vi "PCO_SetApertureF.vi"(8 "error in (no error)":errorcluster {"code" format="%x"}, 9 "dwflagsin":u32, 10 "dwfAperturePos":u32, 11 "hLens":u64) -> (0 "error out":errorcluster {"code" format="%x"}, 1 "dwfAperturePos out":u32, 2 "ErrorMessage":i32 format="%x", 3 "hLens out":u64, 5 "dwflagsout":u32)   [LabVIEW 2019, in "SDK.lvlib" / "LensControl.lvlib"]
doc: "<b>Description:</b>\nSets the current aperture position of the lens control device in f/position * 10 (member of dwApertures)\nPlease select a member of the current dwApertures array.\nThe dwApertures array is reinitialized in case the zoom changes and either PCO_GetApertureF or PCO_SetApertureF are called.\nChange in zoom will be shown in dwflagsout as LENSCONTROL_OUT_ZOOMHASCHANGED.\n\n<b>Supported camera type:</b>\npco.edge CLHS, pco.dimax cs\n\n<b>Descriptor dependency:</b>\nNone"
uses:
  LensControl.lvlib
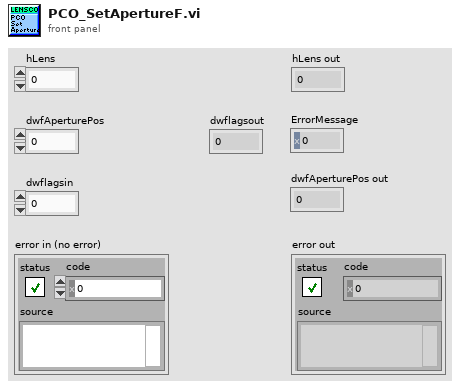
[diagram p1: front panel]
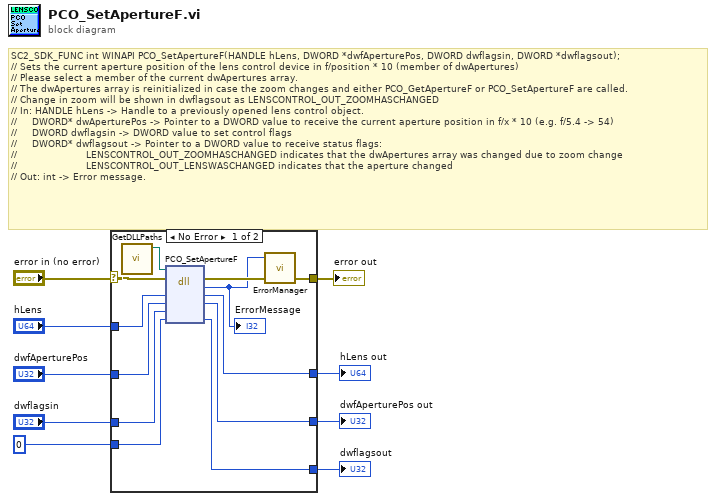
[diagram p0: block diagram]
diagram:
  # "SC2_SDK_FUNC int WINAPI PCO_SetApertureF(HANDLE hLens, DWORD *dwfAperturePos, DWORD dwflagsin, DWORD *dwflagsout);\n// Sets the current aperture position of the lens control device in f/position * 10 (member of dwApertures)\n// Please select a member of the current dwApertures array.\n// The dwApertures array is reinitialized in case the zoom changes and either PCO_GetApertureF or PCO_SetApertureF are called.\n// Change in zoom will be shown in dwflagsout as LENSCONTROL_OUT_ZOOMHASCHANGED\n// In: HANDLE hLens -> Handle to a previously opened lens control object.\n//     DWORD* dwAperturePos -> Pointer to a DWORD value to receive the current aperture position in f/x * 10 (e.g. f/5.4 -> 54)\n//     DWORD dwflagsin -> DWORD value to set control flags\n//     DWORD* dwflagsout -> Pointer to a DWORD value to receive status flags:\n//                       LENSCONTROL_OUT_ZOOMHASCHANGED indicates that the dwApertures array was changed due to zoom change\n//                       LENSCONTROL_OUT_LENSWASCHANGED indicates that the aperture changed\n// Out: int -> Error message."
  n1 = case shown="No Error" "error in (no error)" {
    selector: "error in (no error)" -> [w14 w22]
    tunnel: "hLens" -> [w21 w25]
    tunnel: [w20 w25] -> w8
    tunnel: "dwfAperturePos" -> [w19 w24]
    tunnel: [w18 w24] -> w6
    tunnel: "dwflagsin" -> [w17 _]
    tunnel: u32 0 ("dwflagsout") -> [w16 w23]
    tunnel: [w15 w23] -> w3
    tunnel: [w13 w22] -> w2
    frame No Error {
      n2 = call "GetDLLPaths.vi"() -> ("SC2_Cam_Path"=w10:path)  [unwired: 8 in, 3 out]
      n3 = dll-call lib="?" fn="PCO_SetApertureF"(path in=w10, error in=w14, "hLens"=w21, "dwfAperturePos"=w19, "dwflagsin"=w17, "dwflagsout"=w16) -> (error out=w12:errorcluster, "return type"=w11:i32, "hLens"=w20:u64, "dwfAperturePos"=w18:u32, "dwflagsout"=w15:u32)  [unwired: 2 in, 1 out]
      "ErrorMessage" <- w11
      n4 = call "ErrorManager.vi"("error in (no error)"=w12, "error code"=w11) -> ("error out"=w13:errorcluster)  [unwired: 2 in, 1 out]
    }
    frame Error {
    }
  }
  "hLens out" <- w8
  "dwfAperturePos out" <- w6
  "dwflagsout" <- w3
  "error out" <- w2
